vi "SaveDataPath.vi"() -> (3 "Changed":bool)   [LabVIEW 2013]
doc: "View current datapath and select new."
uses:
  Controls/Enum Save Action Events.ctl
  Globals/DataPathGlobalVariable.vi
  main.lvlib
panel:
  in  "Default":bool
  out "String (transparent)":string caption="Nuværende Mappe"
  in  "DatapathCancelBtn":bool
  in  "DatapathSaveBtn":bool
  in  "DatapathCtrl":path caption="Vælg ny mappe"
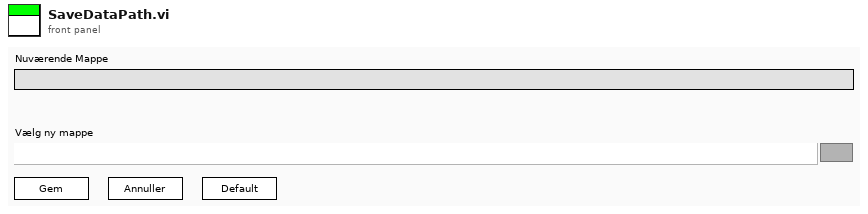
[diagram p1: front panel]
types:
  T1 = typedef "main.lvlib/Enum Save Action Events.ctl" = enum16{"LoadReportPath", "SaveReportPath", "Load Graph Path", "Save Graph Path", "LoadDataPath", "SaveDataPath", "Load Template Path", "Save Template Path", "Load PressureFactor", "Save PressureFactor", "Init", "Load Listbox", "Save Listbox", "LoadHospInfo", "SaveHospInfo", "Load DICOM Activation", "Save DICOM Activation", "LoadDICOMInfoWL", "SaveDICOMInfoWL", "LoadDICOMInfoPACS", "SaveDICOMInfoPACS", "Load ArmCalcMethod", "Save ArmCalcMethod", "LoadItemTags", "SaveItemTags", "LoadDICOMEncoding", "SaveDICOMEncoding", "LoadJournalType", "SaveJournalType", "LoadAcqFilterType", "SaveAcqFilterType", "Load Sequence", "Save Sequence", "Load Acquisition Mode", "Save Acquisition Mode", "Load General Settings", "Save General Settings", "Load Language", "Save Language", "Load Dicom Tags", "Save Dicom Tags", "Load BT Serial", "Save BT Serial", "Load BT License", "Save BT License"}
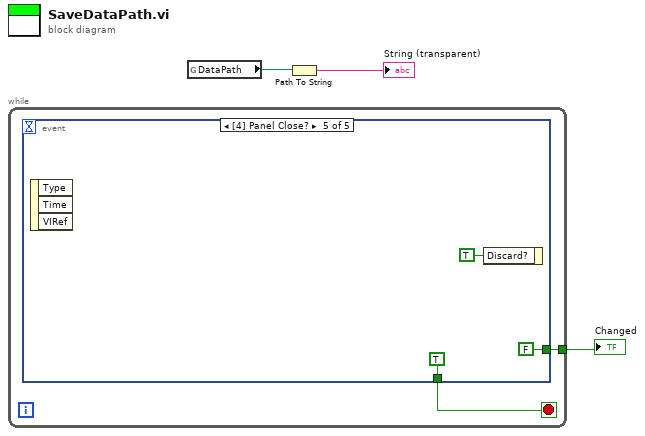
[diagram p0: block diagram]
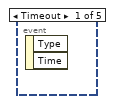
[diagram p2: hidden frame]
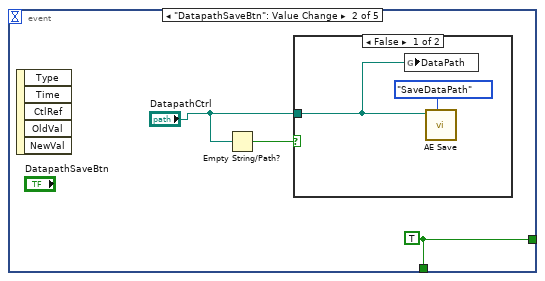
[diagram p3: hidden frame]
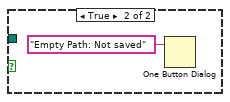
[diagram p4: hidden frame]
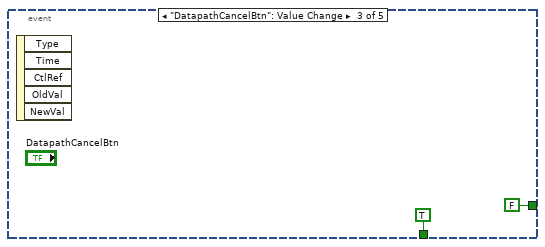
[diagram p5: hidden frame]
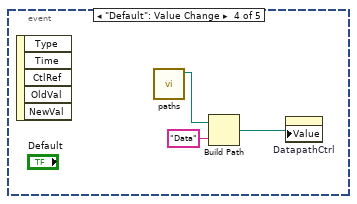
[diagram p6: hidden frame]
diagram:
  n1 = while {
    tunnel: [w4] -> w1
    stop <- w5 stop-if-true
    n2 = event shown="[4] Panel Close?" {
      selector: _ -> [_ _ _ _ _]
      dyn-events: _ -> [_ _ _ _ _]
      timeout: _ -> [_ _ _ _ _]
      tunnel: [_ w6 TRUE ("Changed") _ TRUE ("Changed")] -> w5
      tunnel: [_ w6 FALSE ("Changed") _ FALSE ("Changed")] -> w4
      event Timeout {
        n3 = event-data() -> ()  [unwired: 1 in, 2 out]
      }
      event "DatapathSaveBtn": Value Change {
        w6 = TRUE ("Changed")
        n4 = event-data() -> ()  [unwired: 1 in, 5 out]
        n5 = Empty String/Path?(string/path="DatapathCtrl") -> (empty?=w7:bool)
        n6 = case shown="False" w7 {
          tunnel: "DatapathCtrl" -> [w9 _]
          frame False {
            n7 = global write "DataPathGlobalVariable.vi" "DataPath"(w9) -> ()
            n8 = call "AE Save.vi"("Variant In"=w9, "Action"=Enum_Save_Action_Events."SaveDataPath") -> ()  [unwired: 7 in, 2 out]
          }
          frame True {
            n9 = One Button Dialog(message="Empty Path: Not saved") -> ()  [unwired: 1 in, 1 out]
          }
        }
      }
      event "DatapathCancelBtn": Value Change {
        n10 = event-data() -> ()  [unwired: 1 in, 5 out]
      }
      event "Default": Value Change {
        n11 = event-data() -> ()  [unwired: 1 in, 5 out]
        n12 = call "paths.vi"() -> ("PubAppData"=w14:path)  [unwired: 8 in, 3 out]
        n13 = Build Path(base path=w14, name or relative path="Data") -> (appended path=w16:path)
        n14 = property on="DatapathCtrl" class="Path"("Value"=w16) -> ()  [unwired: 2 in, 2 out]
      }
      event Panel Close? {
        n15 = event-data() -> ()  [unwired: 1 in, 3 out]
        n16 = event-data("Discard?"=TRUE) -> ()  [unwired: 1 in, 1 out]
      }
    }
  }
  "Changed" <- w1
  n17 = global read "DataPathGlobalVariable.vi" "DataPath"() -> (w2:path)
  n18 = Path To String(path=w2) -> (string=→"String (transparent)":string)
